vi "外观.vi"(0 "Data In":T1 caption="数据输入", 2 "Display State In":T3 caption="显示状态输入", 3 "Container State":T4 caption="容器状态") -> (6 "Data Out":T1 caption="数据输出", 7 "Display State Out":T3 caption="显示状态输出", 8 "Action":T2 caption="动作")   [LabVIEW 2014, in "XControl.xctl"]
uses:
  XControl.xctl
  <vilib>/_xctls/Container State.ctl
  <vilib>/_xctls/Action.ctl
  <vilib>/_xctls/XControlSupport.lvlib
panel:
  in  "确定按钮":T1
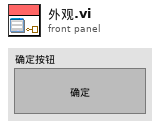
[diagram p1: front panel]
types:
  T1 = typedef "XControl.xctl/数据.ctl" = bool
  T2 = typedef "XControlSupport.lvlib/Action.ctl" = cluster{"Data Changed?":bool, "State Changed?":bool, "Action Name":string}
  T3 = typedef "XControl.xctl/状态.ctl" = cluster{"鼠标进入标题":string, "鼠标离开标题":string}
  T4 = typedef "XControlSupport.lvlib/Container State.ctl" = cluster{"Indicator?":bool, "Run Mode?":bool, " Refnum":refnum<vi>}
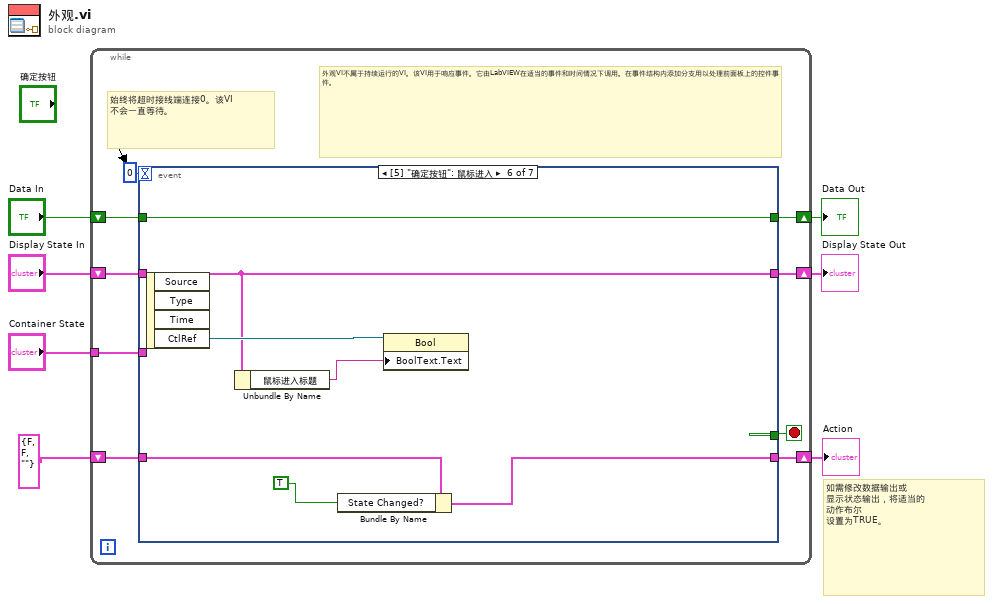
[diagram p0: block diagram]
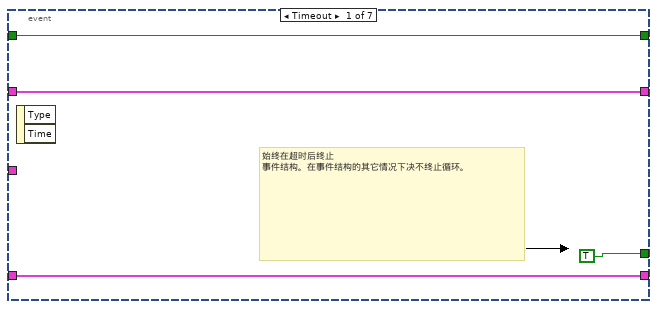
[diagram p2: hidden frame]
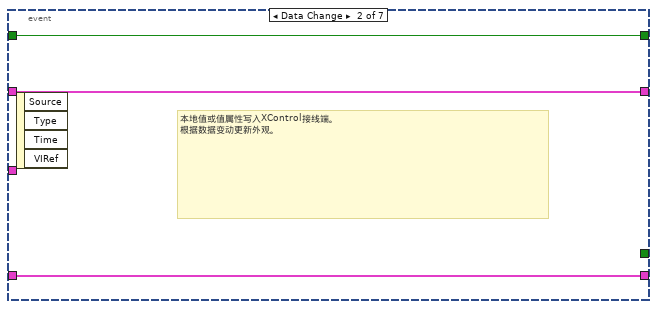
[diagram p3: hidden frame]
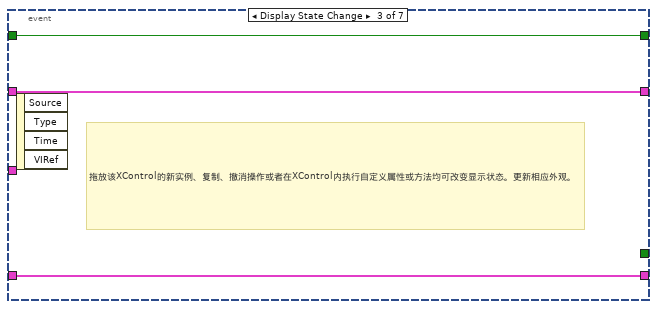
[diagram p4: hidden frame]
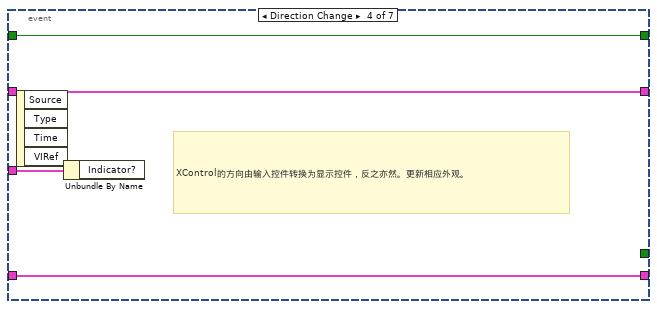
[diagram p5: hidden frame]
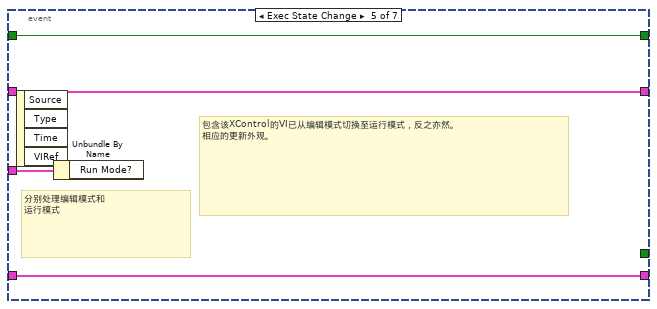
[diagram p6: hidden frame]
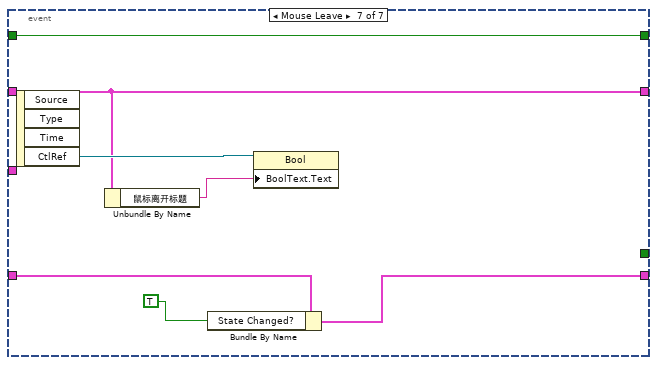
[diagram p7: hidden frame]
diagram:
  # "如需修改数据输出或\n显示状态输出，将适当的\n动作布尔\n设置为TRUE。"
  n1 = while {
    shift-right: [w15] -> w4
    shift-left: "Display State In" -> [w16]
    tunnel: "Container State" -> [w12]
    shift-right: [w10] -> w7
    shift-left: "Data In" -> [w11]
    shift-right: [w8] -> w2
    shift-left: T2 {"Data Changed?"=FALSE, "State Changed?"=FALSE, "Action Name"=""} ("Action") -> [w9]
    stop <- w14 stop-if-true
    # "外观VI不属于持续运行的VI。该VI用于响应事件。它由LabVIEW在适当的事件和时间情况下调用。在事件结构内添加分支用以处理前面板上的控件事件。"
    # "始终将超时接线端连接0。该VI\n不会一直等待。"
    n2 = event shown="[5] \"确定按钮\": 鼠标进入" {
      selector: _ -> [_ _ _ _ _ _ _]
      dyn-events: _ -> [_ _ _ _ _ _ _]
      timeout: 0 -> [_ _ _ _ _ _ _]
      tunnel: w16 -> [w18 w22 w26 w29 w33 w39 w46]
      tunnel: [w18 w22 w26 w29 w33 w39 w46] -> w15
      tunnel: [TRUE _ _ _ _ _ _] -> w14
      tunnel: w12 -> [_ _ _ w30 w34 _ _]
      tunnel: w11 -> [w17 w23 w25 w28 w32 w41 w48]
      tunnel: [w17 w23 w25 w28 w32 w41 w48] -> w10
      tunnel: [w19 w21 w24 w27 w31 w35 w42] -> w8
      tunnel: w9 -> [w19 w21 w24 w27 w31 w36 w43]
      event Timeout {
        # "始终在超时后终止\n事件结构。在事件结构的其它情况下决不终止循环。"
        n3 = event-data() -> ()  [unwired: 1 in, 2 out]
      }
      event Data Change {
        # "本地值或值属性写入XControl接线端。\n根据数据变动更新外观。"
        n4 = event-data() -> ()  [unwired: 1 in, 4 out]
      }
      event Display State Change {
        # "拖放该XControl的新实例、复制、撤消操作或者在XControl内执行自定义属性或方法均可改变显示状态。更新相应外观。"
        n5 = event-data() -> ()  [unwired: 1 in, 4 out]
      }
      event Direction Change {
        # "XControl的方向由输入控件转换为显示控件，反之亦然。更新相应外观。"
        n6 = event-data() -> ()  [unwired: 1 in, 4 out]
        n7 = Unbundle By Name(w30) -> ()  [unwired: 1 out]
      }
      event Exec State Change {
        # "包含该XControl的VI已从编辑模式切换至运行模式，反之亦然。\n相应的更新外观。"
        # "分别处理编辑模式和\n运行模式"
        n8 = event-data() -> ()  [unwired: 1 in, 4 out]
        n9 = Unbundle By Name(w34) -> ()  [unwired: 1 out]
      }
      event Mouse Enter {
        n10 = event-data() -> ("CtlRef"=w40:refnum<vi>)  [unwired: 1 in, 3 out]
        n11 = Unbundle By Name(w39) -> ("鼠标进入标题"=w38:string)
        n12 = Bundle By Name(cluster=w36, "State Changed?"=TRUE) -> (w35:T2)
        n13 = property class="Bool"(reference=w40, "BoolText.Text"=w38) -> ()  [unwired: 1 in, 2 out]
      }
      event Mouse Leave {
        n14 = event-data() -> ("CtlRef"=w47:refnum<vi>)  [unwired: 1 in, 3 out]
        n15 = Unbundle By Name(w46) -> ("鼠标离开标题"=w45:string)
        n16 = Bundle By Name(cluster=w43, "State Changed?"=TRUE) -> (w42:T2)
        n17 = property class="Bool"(reference=w47, "BoolText.Text"=w45) -> ()  [unwired: 1 in, 2 out]
      }
    }
  }
  "Display State Out" <- w4
  "Data Out" <- w7
  "Action" <- w2
